vi "Encoder.vi"(8 "error in (no error)":errorcluster, 9 "Salt 2":string, 10 "Salt 1":string, 11 "Plain Password":string) -> (0 "error out":errorcluster, 3 "Encoded Password":string)   [LabVIEW 2020, in "HTTP Server.lvlib" / "BasicPasswordEncoder.lvclass"]
uses:
  BasicPasswordEncoder.lvclass
  BasicPasswordEncoder.lvclass/BasicPasswordEncoder.ctl
  lv-web-crypto/lv-crypto/Crypto/Hashes/SHA-256/SHA-256.lvclass
  lv-web-crypto/lv-base64/Base64.lvlib
  lv-web-crypto/lv-base64/Variant.ctl
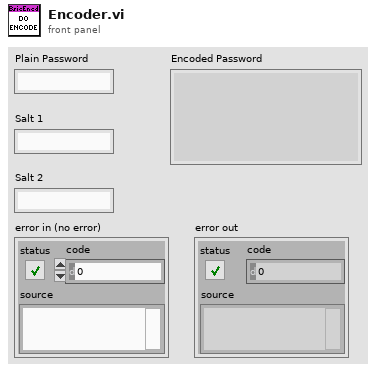
[diagram p1: front panel]
types:
  T1 = typedef "Base64.lvlib/Variant.ctl" = enum16{"Base64", "Base64-URL"}
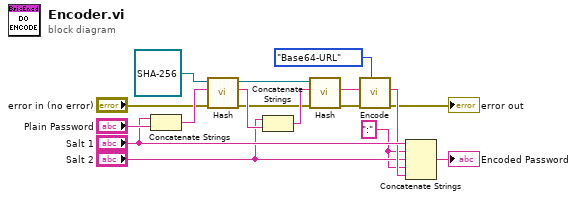
[diagram p0: block diagram]
diagram:
  w6 = ":" ("string")
  n1 = Concatenate Strings("Salt 1", "Plain Password") -> (w15:string)
  n2 = call-dynamic "Hash.vi"("error in (no error)"="error in (no error)", "Message"=w15, "SHA-256 in"=refnum<class "SHA-256.lvclass"> refnum ("Crypto.lvlib:SHA-256.lvclass")) -> ("error out"=w3:errorcluster, "Hash"=w14:string, "SHA-256 out"=w13:refnum<class "SHA-256.lvclass">)  [unwired: 6 in]
  n3 = Concatenate Strings("Salt 2", w14) -> (w12:string)
  n4 = call-dynamic "Hash.vi"("error in (no error)"=w3, "Message"=w12, "SHA-256 in"=w13) -> ("error out"=w2:errorcluster, "Hash"=w10:string)  [unwired: 6 in, 1 out]
  n5 = call "Encode.vi"("Variant (Base64)"=Variant."Base64-URL", "error in (no error)"=w2, "string in (not encoded)"=w10) -> ("error out"=→"error out":errorcluster, "string out (base64-encoded)"=w8:string)  [unwired: 7 in]
  n6 = Concatenate Strings("Salt 1", w6, "Salt 2", w6, w8) -> (→"Encoded Password":string)
